vi "UpdateProfile.vi"(4 "error in":errorcluster, 7 "cluster":T1) -> (0 "error out":errorcluster)   [LabVIEW 2013, in "main.lvlib"]
uses:
  main.lvlib
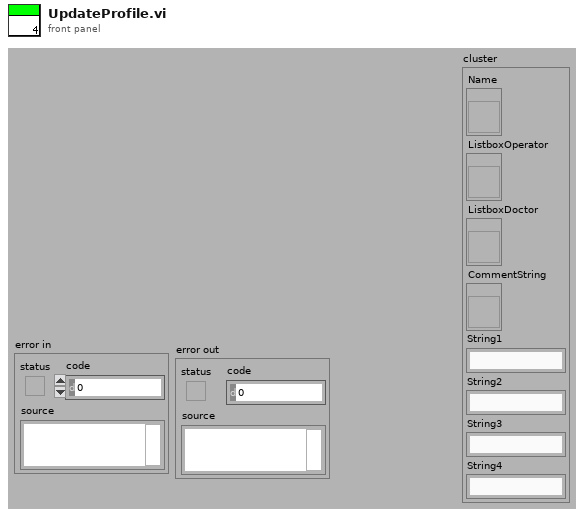
[diagram p1: front panel]
types:
  T1 = cluster{"Name":refnum<vi>, "ListboxOperator":refnum<vi>, "ListboxDoctor":refnum<vi>, "CommentString":refnum<vi>, "String1":string, "String2":string, "String3":string, "String4":string}
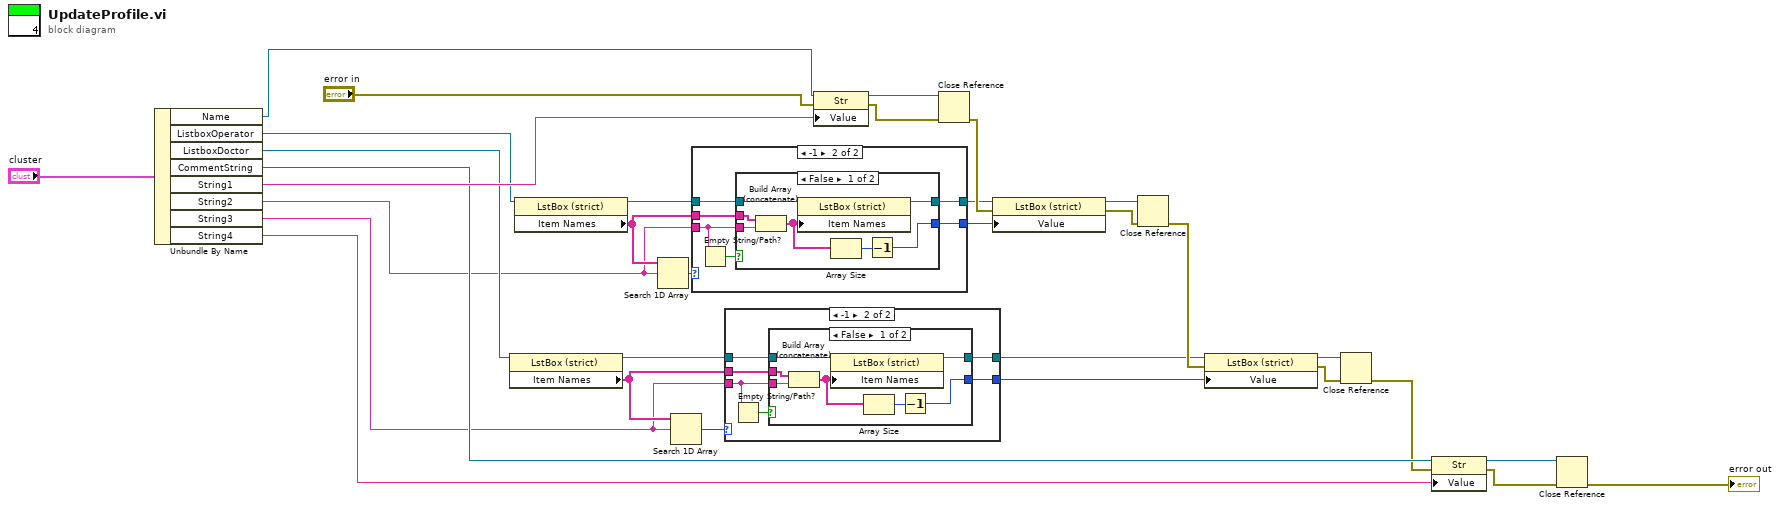
[diagram p0: block diagram]
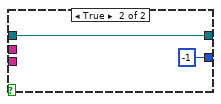
[diagram p3: hidden frame]
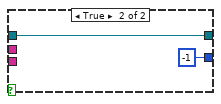
[diagram p5: hidden frame]
diagram:
  n1 = Unbundle By Name("cluster") -> ("Name"=w28:refnum<vi>, "ListboxOperator"=w27:refnum<vi>, "ListboxDoctor"=w26:refnum<vi>, "CommentString"=w25:refnum<vi>, "String1"=w31:string, "String2"=w7:string, "String3"=w1:string, "String4"=w29:string)
  n2 = property class="LstBox (strict)"(reference=w26) -> (reference out=w5:refnum<vi>, "Item Names"=w2:string[])  [unwired: 1 in, 1 out]
  n3 = property class="LstBox (strict)"(reference=w27) -> (reference out=w11:refnum<vi>, "Item Names"=w8:string[])  [unwired: 1 in, 1 out]
  n4 = Search 1D Array(1D array=w8, element=w7) -> (index of element=w12:i32)  [unwired: 1 in]
  n5 = Search 1D Array(1D array=w2, element=w1) -> (index of element=w6:i32)  [unwired: 1 in]
  n6 = case shown="-1" w12 {
    selector: w12 -> [w33 _]
    tunnel: w11 -> [w34 w40]
    tunnel: [w34 w39] -> w10
    tunnel: [w33 w37] -> w9
    tunnel: w8 -> [_ w38]
    tunnel: w7 -> [_ w36]
    frame 0, Default {
    }
    frame -1 {
      n7 = Empty String/Path?(string/path=w36) -> (empty?=w35:bool)
      n8 = case shown="False" w35 {
        tunnel: w40 -> [w47 w49]
        tunnel: [w46 w49] -> w39
        tunnel: w38 -> [w45 _]
        tunnel: w36 -> [w43 _]
        tunnel: [w41 -1] -> w37
        frame False {
          n9 = Build Array (concatenate)(w45, w43) -> (w44:string[])
          n10 = property class="LstBox (strict)"(reference=w47, "Item Names"=w44) -> (reference out=w46:refnum<vi>)  [unwired: 1 in, 1 out]
          n11 = Array Size(array=w44) -> (size(s)=w42:i32)
          n12 = Decrement(x=w42) -> (x-1=w41:i32)
        }
        frame True {
        }
      }
    }
  }
  n13 = case shown="-1" w6 {
    selector: w6 -> [w50 _]
    tunnel: w5 -> [w51 w57]
    tunnel: [w51 w56] -> w4
    tunnel: [w50 w54] -> w3
    tunnel: w2 -> [_ w55]
    tunnel: w1 -> [_ w53]
    frame 0, Default {
    }
    frame -1 {
      n14 = Empty String/Path?(string/path=w53) -> (empty?=w52:bool)
      n15 = case shown="False" w52 {
        tunnel: w57 -> [w64 w66]
        tunnel: [w63 w66] -> w56
        tunnel: w55 -> [w62 _]
        tunnel: w53 -> [w60 _]
        tunnel: [w58 -1] -> w54
        frame False {
          n16 = Build Array (concatenate)(w62, w60) -> (w61:string[])
          n17 = property class="LstBox (strict)"(reference=w64, "Item Names"=w61) -> (reference out=w63:refnum<vi>)  [unwired: 1 in, 1 out]
          n18 = Array Size(array=w61) -> (size(s)=w59:i32)
          n19 = Decrement(x=w59) -> (x-1=w58:i32)
        }
        frame True {
        }
      }
    }
  }
  n20 = property class="Str"(reference=w28, error in="error in", "Value"=w31) -> (reference out=w24:refnum<vi>, error out=w23:errorcluster)
  n21 = Close Reference(reference=w24, error in (no error)=w23) -> (error out=w22:errorcluster)
  n22 = property class="LstBox (strict)"(reference=w10, error in=w22, "Value"=w9) -> (reference out=w21:refnum<vi>, error out=w20:errorcluster)
  n23 = Close Reference(reference=w21, error in (no error)=w20) -> (error out=w19:errorcluster)
  n24 = property class="LstBox (strict)"(reference=w4, error in=w19, "Value"=w3) -> (reference out=w18:refnum<vi>, error out=w17:errorcluster)
  n25 = Close Reference(reference=w18, error in (no error)=w17) -> (error out=w16:errorcluster)
  n26 = property class="Str"(reference=w25, error in=w16, "Value"=w29) -> (reference out=w15:refnum<vi>, error out=w14:errorcluster)
  n27 = Close Reference(reference=w15, error in (no error)=w14) -> (error out=→"error out":errorcluster)
